vi "reportHPForceAndStatus.vi"(0 "ILCCommunications in":refnum<class "ILCCommunications.lvclass">, 5 "HPIndex":i32, 7 "WaitForTrigger":bool, 9 "TriggerIRQ":bool, 11 "error in (no error)":errorcluster) -> (4 "ILCCommunications out":refnum<class "ILCCommunications.lvclass">, 15 "error out":errorcluster)   [LabVIEW 2016, in "ILCCommunications.lvclass"]
uses:
  ILCCommunications.lvclass
  ILCCommunications.lvclass/ILCCommunications.ctl
  Common_RT_Modbus/IModbus/IModbus.lvclass
  Common_RT_HPILC/HPILC/HPILC.lvclass
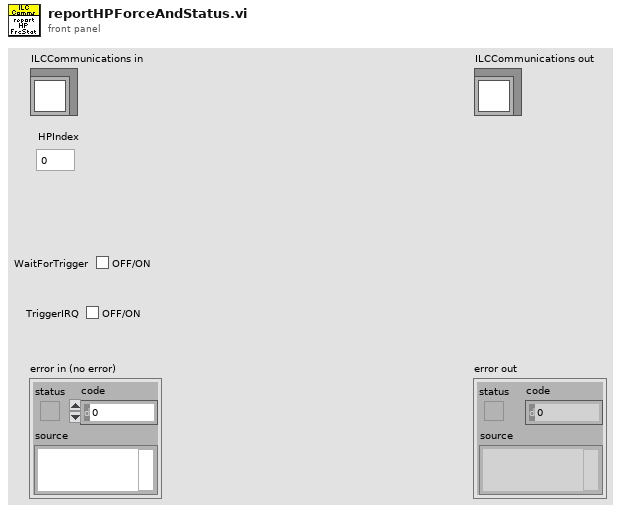
[diagram p1: front panel]
types:
  T1 = typedef "RTModbus.lvlib/TxFrame.ctl" = cluster{"Data":u8[], "WaitForTrigger":bool, "WaitForRx":u16, "TriggerIRQ":bool, "DelayMicroseconds":u16, "DelayMilliseconds":u16, "Timestamp":bool}
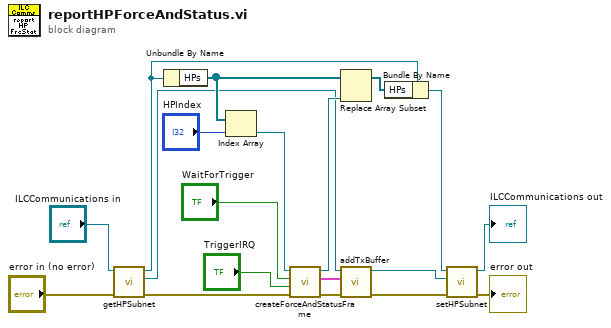
[diagram p0: block diagram]
diagram:
  n1 = call "getHPSubnet.vi"("error in (no error)"="error in (no error)", "ILCCommunications in"="ILCCommunications in") -> ("error out"=w8:errorcluster, "Modbus"=w10:refnum<class "IModbus.lvclass">, "ILCCommunications out"=w5:refnum<class "ILCCommunications.lvclass">)  [unwired: 7 in]
  n2 = Unbundle By Name(w5) -> ("HPs"=w17:refnum<class "HPILC.lvclass">[])
  n3 = Index Array(array=w17, index="HPIndex") -> (element=w12:refnum<class "HPILC.lvclass">)
  n4 = call "createForceAndStatusFrame.vi"("error in (no error)"=w8, "TriggerIRQ"="TriggerIRQ", "WaitForTrigger"="WaitForTrigger", "HPILC in"=w12) -> ("error out"=w13:errorcluster, "TxFrame"=w15:T1, "HPILC out"=w14:refnum<class "HPILC.lvclass">)  [unwired: 5 in]
  n5 = Replace Array Subset(array=w17, new element=w14) -> (w16:refnum<class "HPILC.lvclass">[])  [unwired: 1 in]
  n6 = call-dynamic "addTxBuffer.vi"("error in (no error)"=w13, "TxFrame"=w15, "IModbus in"=w10) -> ("error out"=w7:errorcluster, "IModbus out"=w2:refnum<class "IModbus.lvclass">)  [unwired: 7 in]
  n7 = Bundle By Name(cluster=w5, "HPs"=w16) -> (w3:refnum<class "ILCCommunications.lvclass">)
  n8 = call "setHPSubnet.vi"("error in (no error)"=w7, "Modbus"=w2, "ILCCommunications in"=w3) -> ("error out"=→"error out":errorcluster, "ILCCommunications out"=→"ILCCommunications out":refnum<class "ILCCommunications.lvclass">)  [unwired: 7 in]
